vi "RemovePage.vi"(8 "error in (no error)":errorcluster, 11 "ViewMgr in":refnum<class "ViewMgr.lvclass">) -> (0 "error out":errorcluster, 3 "ViewMgr out":refnum<class "ViewMgr.lvclass">)   [LabVIEW 2020, in "CSM-TagDBDisplayContainer.lvlib" / "ViewMgr.lvclass"]
uses:
  ViewMgr.lvclass
  ViewMgr.lvclass/ViewMgr.ctl
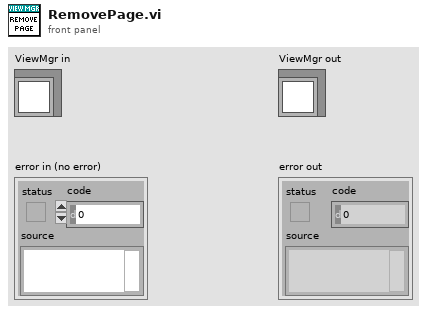
[diagram p1: front panel]
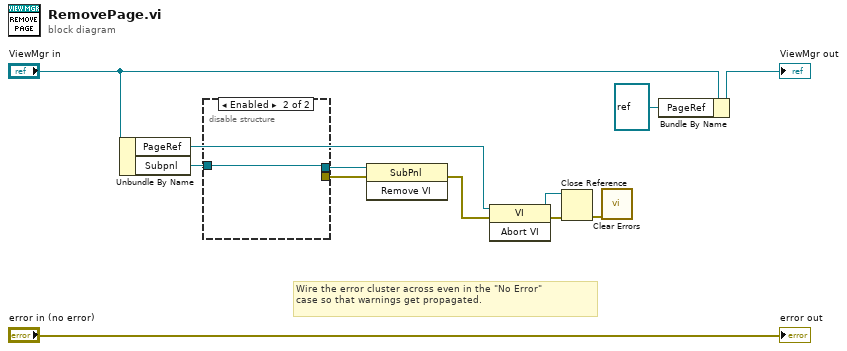
[diagram p0: block diagram]
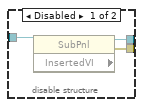
[diagram p2: hidden frame]
diagram:
  # "Wire the error cluster across even in the \"No Error\"\ncase so that warnings get propagated."
  n1 = Unbundle By Name("ViewMgr in") -> ("PageRef"=w1:refnum<vi>, "Subpnl"=w4:refnum<vi>)
  n2 = disable-structure shown="Enabled" {
    disable-tunnel: [w15 _] -> w8
    disable-tunnel: [w14 w16] -> w7
    disable-tunnel: w4 -> [w13 w16]
    frame Disabled {
      n3 = property class="SubPnl" props=["InsertedVI"](reference=w13) -> (reference out=w14:refnum<vi>, error out=w15:errorcluster)  [unwired: 1 in, 1 out]
    }
    frame Enabled {
    }
  }
  n4 = invoke class="SubPnl" method="Remove VI"(reference=w7, error in=w8) -> (error out=w6:errorcluster)  [unwired: 1 in, 2 out]
  n5 = invoke class="VI" method="Abort VI"(reference=w1, error in=w6) -> (reference out=w10:refnum<vi>, error out=w11:errorcluster)  [unwired: 1 in, 1 out]
  n6 = Close Reference(reference=w10, error in (no error)=w11) -> (error out=w9:errorcluster)
  n7 = call <vilib>:"Clear Errors.vi"("error in (no error)"=w9) -> ()  [unwired: 5 in, 2 out]
  n8 = Bundle By Name(cluster="ViewMgr in", "PageRef"=refnum<vi> refnum) -> (→"ViewMgr out":refnum<class "ViewMgr.lvclass">)
  "error out" <- "error in (no error)"
